vi "_session_set_data.vi"(8 "error in":errorcluster caption="error in (no error)", 10 "Session User Data in":T1={"IDN string"="", "Instrument FW"="", "Instr type"="", "Instr type for err. msg."="", "Installed Options"=[], "Ignore Error Messages"="", "Logging params"=variant, "OPC Timeout"=5000, "VISA Timeout"=10000, "STB Poll VISA Timeout"=5000, "Additional Flags"=4, "Wait Before Read"=0, "Wait Before Write"=0, "Option String Flags"=0, "IO Segment Size"=10000000, "VISA Access Mode"=4, "Interface Type"=enum."TCPIP", "OPC Wait Mode"=enum."STBpolling", "Bin Float Number  Format"=enum."Float_4_Bytes_Swapped", "Bin Integer Number Format"=enum."Int32_4_Bytes_Swapped", "Simulate"=FALSE, "VXIcapable"=TRUE, "Duplicate Session"=FALSE, "Add LF to Write"=TRUE, "Logging"=FALSE, "Fast Sweep"=FALSE, "Query Instrument Status"=TRUE, "Check Range"=TRUE, "Check Options"=TRUE} {"VISA Access Mode" items=["VISA Defaults"=0, "Exclusive Lock"=1, "Load Settings"=4]; "IO Segment Size" format="%#.6p"; "Additional Flags" format="%011b"}, 11 "VISA resource name":refnum<visa-resource-name>) -> (0 "error out":errorcluster, 3 "VISA resource name out":refnum<visa-resource-name>)   [LabVIEW 2022 SP3, in "hmp4000_rsidr_core.lvlib"]
uses:
  hmp4000_rsidr_core.lvlib
  type_Session_Data.ctl
  type_VisaAccessMode.ctl
  type_InterfaceType.ctl
  type_OPC_Wait_Mode.ctl
  type_Binary_Float_Number_Format.ctl
  type_Binary_Integer_Number_Format.ctl
  _type_Operation_Fgv_Session.ctl
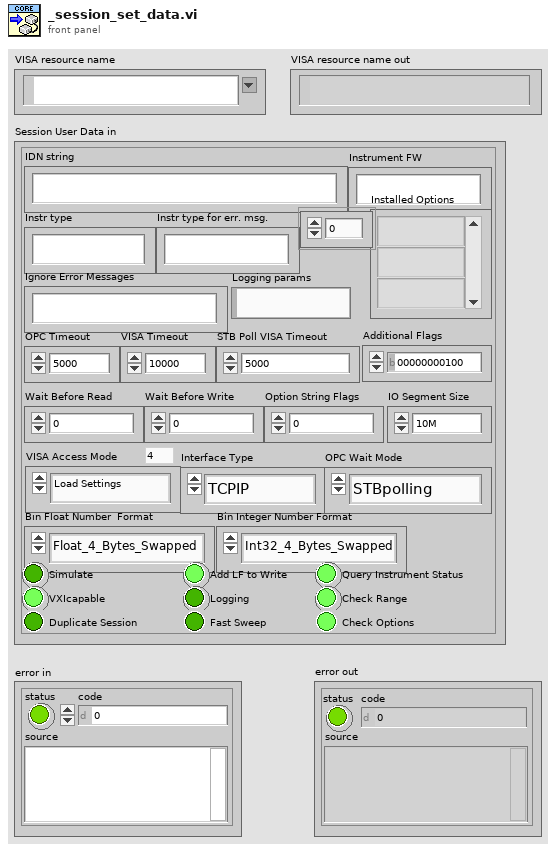
[diagram p1: front panel]
types:
  T1 = typedef "hmp4000_rsidr_core.lvlib/type_Session_Data.ctl" = cluster{"IDN string":string, "Instrument FW":string, "Instr type":string, "Instr type for err. msg.":string, "Installed Options":string[], "Ignore Error Messages":string, "Logging params":variant, "OPC Timeout":i32, "VISA Timeout":i32, "STB Poll VISA Timeout":i32, "Additional Flags":i32, "Wait Before Read":i32, "Wait Before Write":i32, "Option String Flags":i32, "IO Segment Size":i64, "VISA Access Mode":T2, "Interface Type":T3, "OPC Wait Mode":T4, "Bin Float Number  Format":T5, "Bin Integer Number Format":T6, "Simulate":bool, "VXIcapable":bool, "Duplicate Session":bool, "Add LF to Write":bool, "Logging":bool, "Fast Sweep":bool, "Query Instrument Status":bool, "Check Range":bool, "Check Options":bool}
  T2 = typedef "hmp4000_rsidr_core.lvlib/type_VisaAccessMode.ctl" = u16
  T3 = typedef "hmp4000_rsidr_core.lvlib/type_InterfaceType.ctl" = enum16{"Unknown", "GPIB", "VXI", "GPIB_VXI", "ASRL", "PXI", "TCPIP", "USB", "SOCKET"}
  T4 = typedef "hmp4000_rsidr_core.lvlib/type_OPC_Wait_Mode.ctl" = enum16{"STBpolling", "STBpollingSlow", "STBpollingSuperSlow", "ServiceRequest", "OPCquery"}
  T5 = typedef "hmp4000_rsidr_core.lvlib/type_Binary_Float_Number_Format.ctl" = enum16{"Float_4_Bytes_Swapped", "Float_4_Bytes", "Double_8_Bytes_Swapped", "Double_8_Bytes"}
  T6 = typedef "hmp4000_rsidr_core.lvlib/type_Binary_Integer_Number_Format.ctl" = enum16{"Int32_4_Bytes_Swapped", "Int32_4 Bytes", "Int16_2_Bytes_Swapped", "Int16_2_Bytes"}
  T7 = typedef "hmp4000_rsidr_core.lvlib/_type_Operation_Fgv_Session.ctl" = enum16{"Initialize", "GetData", "SetData", "Clear", "GetSessionIx"}
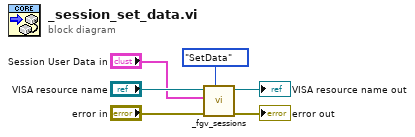
[diagram p0: block diagram]
diagram:
  n1 = call "_fgv_sessions.vi"("Operation"=_type_Operation_Fgv_Session."SetData", "error in"="error in", "Session User Data in (None)"="Session User Data in", "VISA resource name"="VISA resource name") -> ("error out"=→"error out":errorcluster, "VISA resource name out"=→"VISA resource name out":refnum<visa-resource-name>)  [unwired: 4 in, 2 out]
